vi "niRFUtil RFHS Channelizer ChannelizerRead CSG.vi"(0 "Channelizer Ref":refnum<data-value>, 1 "Read Mode":T2, 2 "Benchmark Task":T1, 7 "Length":i32=-1, 9 "Channnel":i32, 11 "error in (no error)":errorcluster) -> (4 "Channelizer Ref (out)":refnum<data-value>, 6 "Channel Data":csg[](array[numeric]), 15 "error out":errorcluster)   [LabVIEW 2015, in "niRFUtil.lvlib"]
uses:
  niRFUtil.lvlib
  Includes/niRFUtil RFHS Channelizer ChannelizerInfo CSG.ctl
  Includes/niRFUtil RFHS Channelizer FilterRef.ctl
  Includes/niRFUtil RFHS Channelizer ChannelizerBufferingMode.ctl
  Utilities/Data FIFO/niRFUtil RFHS FIFO Reference.ctl
  Utilities/Data FIFO/niRFUtil RFHS FIFO.ctl
  Includes/niRFUtil RFHS Channelizer ChannelizerType.ctl
  Includes/niRFUtil RFHS Channelizer ChannelizerFlags.ctl
  Includes/niRFUtil RFHS Channelizer ChannelizerReadMode CSG.ctl
  Utilities/Benchmark/niRFUtil RFHS Benchmark Task.ctl
  Includes/niRFUtil RFHS Channelizer Ref.ctl
  Includes/niRFUtil RFHS Channelizer ChannelizerErrors.ctl
  Utilities/niRFUtil RFHS Util Dll Path.vi
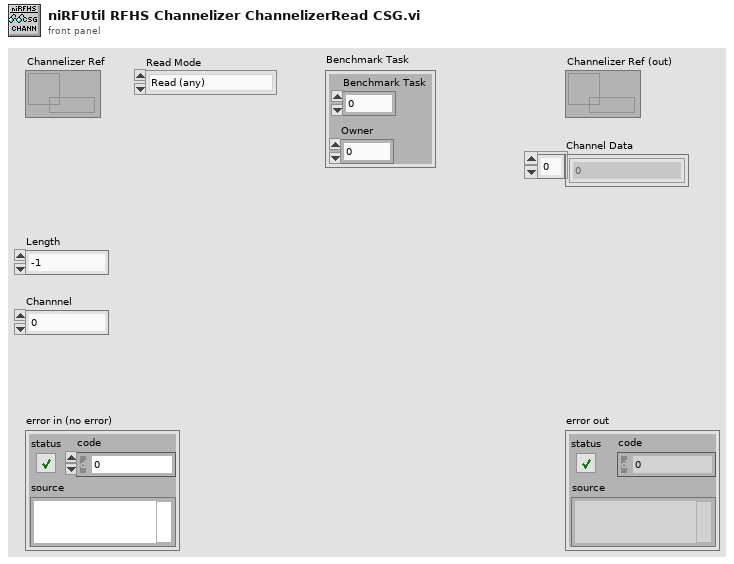
[diagram p1: front panel]
types:
  T1 = typedef "niRFUtil.lvlib/niRFUtil RFHS Benchmark Task.ctl" = cluster{"Benchmark Task":u64, "Owner":u32}
  T2 = typedef "niRFUtil.lvlib/niRFUtil RFHS Channelizer ChannelizerReadMode CSG.ctl" = enum16{"Read (any)", "Read (exact)", "Peek (any)", "Peek (exact)"}
  T3 = typedef "niRFUtil.lvlib/niRFUtil RFHS Channelizer Ref.ctl" = refnum<data-value>
  T4 = typedef "niRFUtil.lvlib/niRFUtil RFHS Channelizer ChannelizerErrors.ctl" = enum32{"No Error", "Invalid Channel", "Internal Error", "Invalid Channel fs", "Invalid Phase Shift", "Invalid fs", "Invalid Number Of Channles", "Invalid FFT Channel fs", "Invalid Resampler Channel fs", "Not a 15kHz Multiple", "Invalid Channel fc", "Invalid passBW/stopBW", "Coerced Rejection", "Requires Internal Buffer", "Duplicated Destination Channel Name", "Configuration Format Error", "Illegal Execution state", "DLL not found", "DLL loading failure", "AVX instruction failure"}
  T5 = typedef "niRFUtil.lvlib/niRFUtil RFHS Channelizer ChannelizerInfo CSG.ctl" = cluster{"Filter LVRef":T6, "Mode":T7, "History":csg[], "Buffer":csg[], "FIFO":T8, "History Len":u32, "Float Cache":csg[], "Double Cache":cdb[], "Type":T10, "Resample Phase":dbl, "fft1Descriptors":u64[], "fft2Descriptors":u64[], "FFT tBuf":csg[], "guardBandLen":i32, "FFT History":csg[], "FFT History Len":u32, "FFTInitDone":u32, "FFT Filter LVRefs":T6[], "FFT fc Offs":u32[], "fft2Sizes":u32[], "BufferW":u32[], "BufferR":u32[], "Buff Off":u32[], "Phase0 (fshift)":dbl[], "Phase (fshift)":dbl[], "fs phase step":dbl[], "Resample Step":dbl, "Flags":T11, "Reset Cnt":i64, "Filter Pass":u32, "Stages":variant[]}
  T6 = typedef "niRFUtil.lvlib/niRFUtil RFHS Channelizer FilterRef.ctl" = cluster{"Ref":u64, "GUID":u64, "Upsample":i32, "Downsample":i32, "Size":i32, "Num Taps":i32}
  T7 = typedef "niRFUtil.lvlib/niRFUtil RFHS Channelizer ChannelizerBufferingMode.ctl" = enum32{"Unbuffered", "Finite", "Continuous"}
  T8 = typedef "niRFUtil.lvlib/niRFUtil RFHS FIFO Reference.ctl" = cluster{"Read Lock":refnum<data-value>, "Info":T9, "Write Lock":refnum<data-value>}
  T9 = typedef "niRFUtil.lvlib/niRFUtil RFHS FIFO.ctl" = cluster{"ID":u64, "Length":u32}
  T10 = typedef "niRFUtil.lvlib/niRFUtil RFHS Channelizer ChannelizerType.ctl" = enum32{"Auto", "Frequency Shift Only", "Resampler Only"}
  T11 = typedef "niRFUtil.lvlib/niRFUtil RFHS Channelizer ChannelizerFlags.ctl" = u32
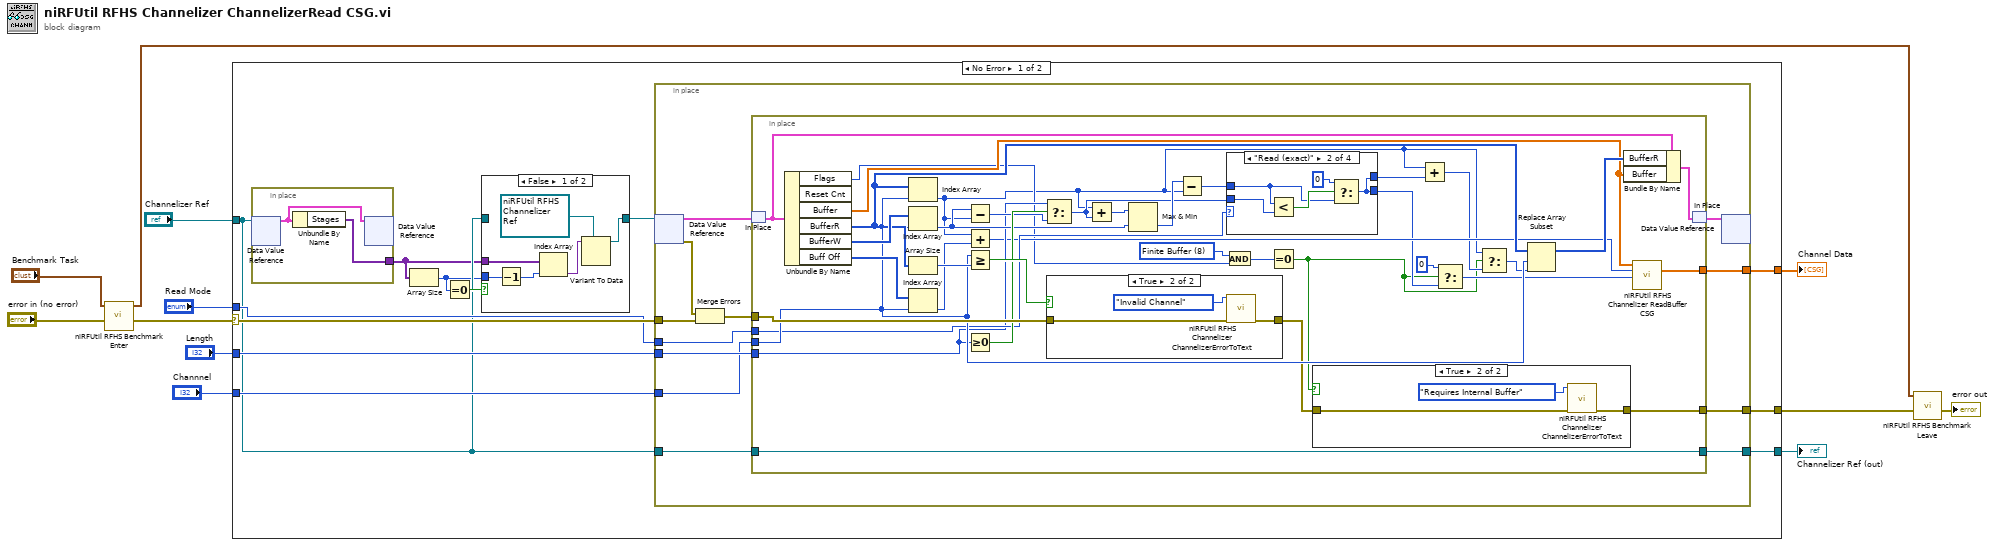
[diagram p0: block diagram]
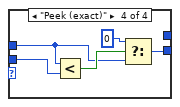
[diagram p6: hidden frame]
diagram:
  n1 = call "niRFUtil RFHS Benchmark Enter.vi"("error in (no error)"="error in (no error)", "Benchmark Task (Parent)"="Benchmark Task") -> ("error out"=w10:errorcluster, "Benchmark Task (Self)"=w5:T1)  [unwired: 8 in]
  n2 = case shown="No Error" w10 {
    selector: w10 -> [w24 w104]
    tunnel: [w23 w104] -> w11
    tunnel: [w22 _] -> w8
    tunnel: "Channelizer Ref" -> [w15 w103]
    tunnel: [w21 w103] -> w6
    tunnel: "Length" -> [w20 _]
    tunnel: "Channnel" -> [w19 _]
    tunnel: "Read Mode" -> [w18 _]
    frame No Error {
      n3 = in-place {
        in-place-border: [w32] -> w14
        n4 = in-place-dvr #1(w15) -> (w33:T5)  [unwired: 1 out]
        n5 = Unbundle By Name(w33) -> ("Stages"=w32:variant[])
        n6 = in-place-dvr #1(w33) -> ()  [unwired: 2 out]
      }
      n7 = Array Size(array=w14) -> (size(s)=w13:i32)
      n8 = Equal To 0?(x=w13) -> (x = 0?=w17:bool)
      n9 = case shown="False" w17 {
        tunnel: [w25 w31] -> w16
        tunnel: w15 -> [_ w31]
        tunnel: w14 -> [w29 _]
        tunnel: w13 -> [w28 _]
        frame False {
          n10 = Decrement(x=w28) -> (x-1=w30:i32)
          n11 = Index Array(array=w29, index=w30) -> (element=w27:variant)
          n12 = Variant To Data(type=T3 refnum ("Channelizer Ref"), Variant=w27) -> (data=w25:T3)  [unwired: 1 in, 1 out]
        }
        frame True {
        }
      }
      n13 = in-place {
        in-place-border: w24 -> [w38]
        in-place-border: [w42] -> w23
        in-place-border: [w43] -> w22
        in-place-border: w15 -> [w45]
        in-place-border: [w44] -> w21
        in-place-border: w20 -> [w41]
        in-place-border: w19 -> [w36]
        in-place-border: w18 -> [w35]
        n14 = in-place-dvr #2(w16) -> (w34:T5, w39:errorcluster)
        n15 = Merge Errors(w39, w38) -> (w37:errorcluster)
        n16 = in-place {
          in-place-border: w45 -> [w65]
          in-place-border: w37 -> [w74]
          in-place-border: [w65] -> w44
          in-place-border: [w63] -> w43
          in-place-border: [w47] -> w42
          in-place-border: w41 -> [w61]
          in-place-border: w36 -> [w66]
          in-place-border: w35 -> [w62]
          w57 = T11 8 items=["None"=0, "Skip Stage 1"=1, "FFT Stage"=2, "Frequency Shift"=4, "Finite Buffer"=8, "Reset"=16, "Input Len Estimate"=32, "C buffers"=64, "Input From Ref"=128] ("Flags")
          n17 = in-place-match #3(w34) -> (w81:T5)
          n18 = Unbundle By Name(w81) -> ("Flags"=w56:T11, "Buffer"=w64:csg[], "BufferR"=w77:u32[], "BufferW"=w82:u32[], "Buff Off"=w78:u32[])  [unwired: 1 out]
          n19 = Index Array(array=w77, index=w66) -> (element=w53:u32)
          n20 = Index Array(array=w82, index=w66) -> (element=w69:u32)
          n21 = Array Size(array=w77) -> (size(s)=w76:i32)
          n22 = Index Array(array=w78, index=w66) -> (element=w68:u32)
          n23 = Subtract(x=w69, y=w53) -> (x-y=w70:u32)
          n24 = Add(x=w53, y=w68) -> (x+y=w60:u32)
          n25 = Greater Or Equal?(x=w66, y=w76) -> (x >= y?=w75:bool)
          n26 = Greater Or Equal To 0?(x=w61) -> (x >= 0?=w71:bool)
          n27 = Select(t=w61, s=w71, f=w70) -> (s? t:f=w58:u32)
          n28 = case shown="True" w75 {
            tunnel: w74 -> [w99 w101]
            tunnel: [w99 w100] -> w48
            frame False {
            }
            frame True {
              n29 = call "niRFUtil RFHS Channelizer ChannelizerErrorToText.vi"("Error List"=niRFUtil_RFHS_Channelizer_ChannelizerErrors."Invalid Channel", "error in (no error)"=w101) -> ("error out"=w100:errorcluster)  [unwired: 13 in]
            }
          }
          n30 = Add(x=w53, y=w58) -> (x+y=w73:u32)
          n31 = Max & Min(x=w73, y=w69) -> (min(x,y)=w67:u32)  [unwired: 1 out]
          n32 = Subtract(x=w67, y=w53) -> (x-y=w72:u32)
          n33 = And(x=w57, y=w56) -> (x .and. y?=w55:T11)
          n34 = case shown="\"Read (exact)\"" w62 {
            tunnel: w72 -> [w87 w90 w93 w96]
            tunnel: [w87 w88 w93 w94] -> w51
            tunnel: w58 -> [_ w92 _ w98]
            tunnel: [w87 w88 _ _] -> w59
            frame "Read (any)" {
            }
            frame "Read (exact)" {
              n35 = Less?(x=w90, y=w92) -> (x < y?=w91:bool)
              n36 = Select(t=u32 0, s=w91, f=w90) -> (s? t:f=w88:u32)
            }
            frame "Peek (any)" {
            }
            frame "Peek (exact)" {
              n37 = Less?(x=w96, y=w98) -> (x < y?=w97:bool)
              n38 = Select(t=u32 0, s=w97, f=w96) -> (s? t:f=w94:u32)
            }
          }
          n39 = Equal To 0?(x=w55) -> (x = 0?=w46:bool)
          n40 = case shown="True" w46 {
            tunnel: w48 -> [w83 w85]
            tunnel: [w83 w84] -> w47
            frame False {
            }
            frame True {
              n41 = call "niRFUtil RFHS Channelizer ChannelizerErrorToText.vi"("Error List"=niRFUtil_RFHS_Channelizer_ChannelizerErrors."Requires Internal Buffer", "error in (no error)"=w85) -> ("error out"=w84:errorcluster)  [unwired: 13 in]
            }
          }
          n42 = Add(x=w53, y=w59) -> (x+y=w54:u32)
          n43 = Select(t=u32 0, s=w46, f=w51) -> (s? t:f=w49:u32)
          n44 = Select(t=w53, s=w46, f=w54) -> (s? t:f=w52:u32)
          n45 = Replace Array Subset(array=w77, new element=w52, index=w66) -> (w79:u32[])
          n46 = Bundle By Name(cluster=w81, "BufferR"=w79, "Buffer"=w64) -> (w80:T5)
          n47 = call "niRFUtil RFHS Channelizer ReadBuffer CSG.vi"("Buffer"=w64, "Index"=w60, "Length"=w49) -> ("Data"=w63:csg[])  [unwired: 12 in]
          n48 = in-place-match #3(w80) -> (w40:T5)
        }
        n49 = in-place-dvr #2(w40) -> ()  [unwired: 2 out]
      }
    }
    frame Error {
    }
  }
  "Channel Data" <- w8
  "Channelizer Ref (out)" <- w6
  n50 = call "niRFUtil RFHS Benchmark Leave.vi"("error in (no error)"=w11, "Benchmark Task Self"=w5) -> ("error out"=→"error out":errorcluster)  [unwired: 8 in, 1 out]
